vi "StdErr1.vi"(11 "2D Array":u64[][](array[numeric]) format="%.1f") -> (0 "Deviation by row":dbl[][](array[numeric]) format="%.2f", 1 "STD":dbl[](array[numeric]) format="%#_3g", 2 "Variance":dbl[](array[numeric]) format="%#_4g", 3 "Average by row":u64[](array[numeric]) format="%-2.1f", 4 "Mean as number":dbl format="%#_3g")   [LabVIEW 2023]
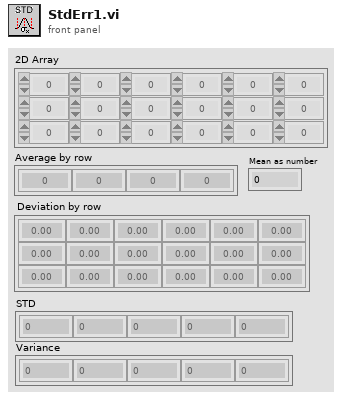
[diagram p1: front panel]
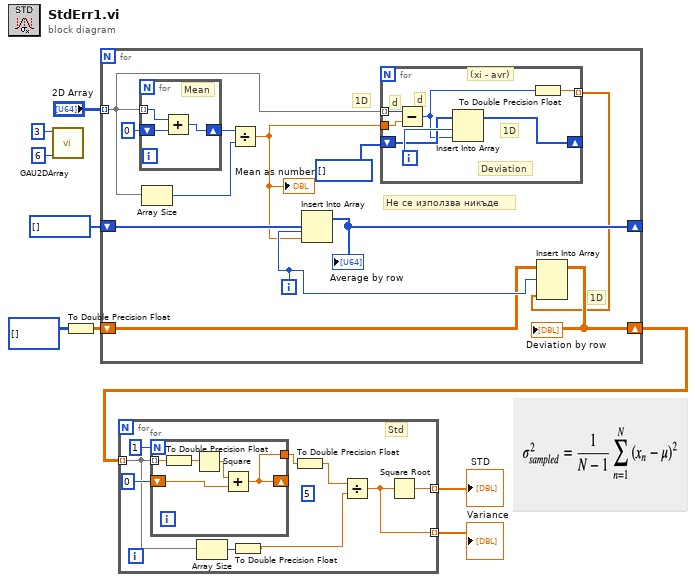
[diagram p0: block diagram]
diagram:
  n1 = call "GAU2DArray.vi"("Colums"=6, "Rows"=3) -> ()  [unwired: 8 in, 2 out]
  n2 = To Double Precision Float(number=i64[][] []) -> (double precision float=w1:dbl[][])
  n3 = for {
    tunnel: "2D Array" -> [w12] mode=indexing
    shift-right: [w17] -> _
    shift-left: u64[] [] -> [w20]
    shift-right: [w14] -> w5
    shift-left: w1 -> [w15]
    i -> [w16]
    # "Не се използва никъде"
    # "1D"
    # "1D"
    n4 = for {
      tunnel: w12 -> [w31] mode=indexing
      shift-right: [w30] -> w19
      shift-left: 0 -> [w29]
      # "Mean"
      n5 = Add(x=w31, y=w29) -> (x+y=w30:u64)
    }
    n6 = Array Size(array=w12) -> (size(s)=w10:i32)
    n7 = Divide(x=w19, y=w10) -> (x/y=w13:dbl)
    "Mean as number" <- w13
    n8 = Insert Into Array(array=w20, index=w16, new element=w13) -> (w17:u64[])
    "Average by row" <- w17
    n9 = for {
      tunnel: w12 -> [w28] mode=indexing
      tunnel: w13 -> [w27]
      shift-right: [w24] -> _
      shift-left: u64[] [] -> [w25]
      tunnel: [w22] -> w11 mode=indexing
      i -> [w26]
      # "(xi - avr)"
      # "d"
      # "d"
      # "1D"
      # "Deviation"
      n10 = Subtract(x=w28, y=w27) -> (x-y=w23:i64)
      n11 = Insert Into Array "Insert Into Array"(array=w25, index=w26, new element=w23) -> (w24:u64[])
      n12 = To Double Precision Float(number=w23) -> (double precision float=w22:dbl)
    }
    n13 = Insert Into Array "Insert Into Array"(array=w15, index (row)=w16, new element=w11) -> (w14:dbl[][])  [unwired: 1 in]
    "Deviation by row" <- w14
  }
  n14 = for {
    tunnel: w5 -> [w34] mode=indexing
    tunnel: [w39] -> w4 mode=indexing
    tunnel: [w38] -> w3 mode=indexing
    (unwired) i64 5 ("y")
    # "Std"
    n15 = for {
      N: 1 -> [_]
      tunnel: w34 -> [w42] mode=indexing
      shift-right: [w41] -> _
      shift-left: i64 0 -> [w44]
      tunnel: [w41] -> w35
      n16 = To Double Precision Float(number=w42) -> (double precision float=w43:dbl)
      n17 = Square(x=w43) -> (x^2=w45:dbl)
      n18 = Add(x=w45, y=w44) -> (x+y=w41:dbl)
    }
    n19 = Array Size(array=w34) -> (size(s)=w33:i32)
    n20 = To Double Precision Float(number=w33) -> (double precision float=w32:dbl)
    n21 = To Double Precision Float(number=w35) -> (double precision float=w36:dbl)
    n22 = Divide(x=w36, y=w32) -> (x/y=w38:dbl)
    n23 = Square Root(x=w38) -> (sqrt(x)=w39:dbl)
  }
  "STD" <- w4
  "Variance" <- w3
